vi "PSDOM_DMG_Get Ctrl Label.vi"(10 "Label":string) -> (2 "InCluster?":bool, 4 "Ctrl Label":string)   [LabVIEW 2013]
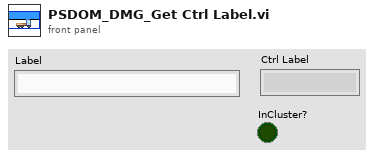
[diagram p1: front panel]
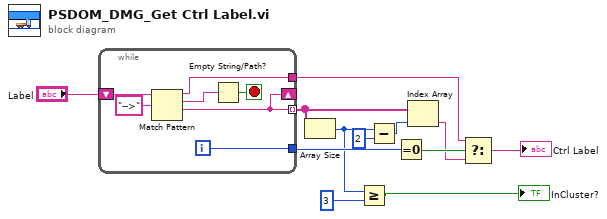
[diagram p0: block diagram]
diagram:
  n1 = while {
    shift-right: [w15] -> _
    shift-left: "Label" -> [w18]
    tunnel: [w15] -> w11 mode=indexing
    tunnel: [w14] -> w8
    tunnel: [w13] -> w6
    i -> [w14]
    stop <- w16 stop-if-true
    n2 = Match Pattern(string=w18, regular expression="-->" ("正则表达式")) -> (before substring=w13:string, match substring=w17:string, after substring=w15:string)  [unwired: 1 in, 1 out]
    n3 = Empty String/Path?(string/path=w17) -> (empty?=w16:bool)
  }
  n4 = Array Size(array=w11) -> (size(s)=w3:i32)
  n5 = Greater Or Equal?(x=w3, y=3) -> (x >= y?=→"InCluster?":bool)
  n6 = Subtract(x=w3, y=2) -> (x-y=w10:i32)
  n7 = Equal To 0?(x=w8) -> (x = 0?=w7:bool)
  n8 = Index Array(array=w11, index=w10) -> (element=w5:string)
  n9 = Select(t=w6, s=w7, f=w5) -> (s? t:f=→"Ctrl Label":string)
